vi "Get Array Data Variant.vi"(8 "error in (no error)":errorcluster, 11 "Core Threads Configuration in":refnum<class "Core Threads Configuration.lvclass">) -> (0 "error out":errorcluster, 1 "data version":T1, 2 "data":variant, 3 "Core Threads Configuration out":refnum<class "Core Threads Configuration.lvclass">)   [LabVIEW 2017, in "DSF Core.lvlib" / "Core Threads Configuration.lvclass"]
uses:
  Core Threads Configuration.lvclass
  C:/Git/DSF/Core/Classes/Configuration/Configuration.lvclass
  Typedefs/DSF Version Info.ctl
  Configuration.lvclass
  DSF Core.lvlib
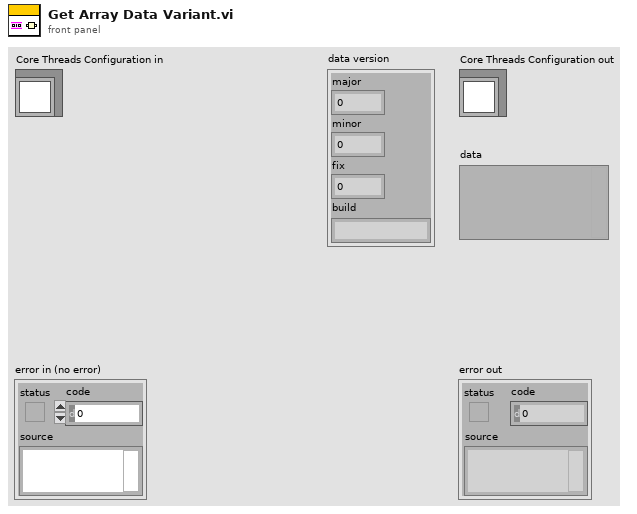
[diagram p1: front panel]
types:
  T1 = typedef "DSF Core.lvlib/DSF Version Info.ctl" = cluster{"major":i32, "minor":i32, "fix":i32, "build":string}
  T2 = typedef "DSF Core.lvlib/Core Threads Configuration.lvclass/Configuration.ctl" = cluster{"processor":i32, "priority offset":i16}
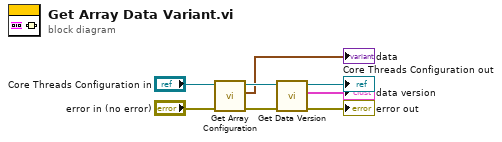
[diagram p0: block diagram]
diagram:
  n1 = call "Get Array Configuration.vi"("error in (no error)"="error in (no error)", "Core Threads Configuration in"="Core Threads Configuration in") -> ("error out"=w6:errorcluster, "thread configurations"=→"data":T2[], "Core Threads Configuration out"=w3:refnum<class "Core Threads Configuration.lvclass">)  [unwired: 7 in]
  n2 = call "Get Data Version.vi"("error in (no error)"=w6, "Configuration in"=w3) -> ("error out"=→"error out":errorcluster, "data version"=→"data version":T1, "Configuration out"=→"Core Threads Configuration out":refnum<class "Core Threads Configuration.lvclass">)  [unwired: 7 in]
